vi "KE622x -- Get Buf Size.vi"(0 "Resource In":refnum<visa-resource-name>, 1 "Check For SCPI Errors? (T)":bool=TRUE, 11 "error in (no error)":errorcluster) -> (4 "Resource Out (dupl)":refnum<visa-resource-name>, 8 "Buffer Size (Num Readings)":T1 min=1 max=65536 step=1, 15 "error out":errorcluster)   [LabVIEW 2019, in "Keithley 622x.lvlib"]
uses:
  Keithley 622x.lvlib
  Typedefs/KE622x -- Trace Buf Size.ctl
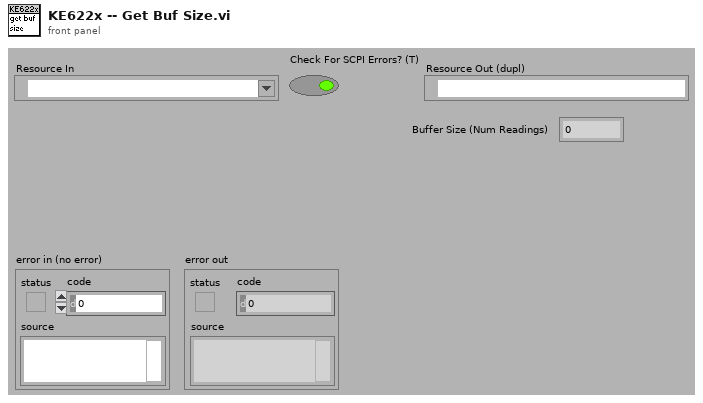
[diagram p1: front panel]
types:
  T1 = typedef "Keithley 622x.lvlib/KE622x -- Trace Buf Size.ctl" = u32
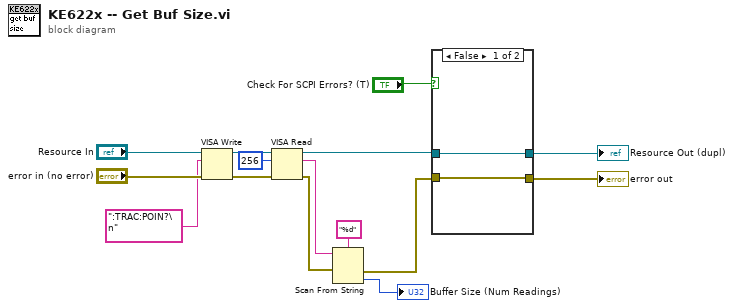
[diagram p0: block diagram]
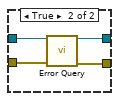
[diagram p2: hidden frame]
diagram:
  n1 = VISA Write(VISA resource name="Resource In", write buffer=":TRAC:POIN?\n" ("format string"), error in (no error)="error in (no error)") -> (VISA resource name out=w15:refnum<visa-resource-name>, error out=w14:errorcluster)  [unwired: 1 out]
  n2 = VISA Read(VISA resource name=w15, byte count=u32 256, error in (no error)=w14) -> (VISA resource name out=w5:refnum<visa-resource-name>, read buffer=w9:string, error out=w7:errorcluster)  [unwired: 1 out]
  n3 = Scan From String(format string="%d", input string=w9, error in=w7) -> (error out=w6:errorcluster, output 1=→"Buffer Size (Num Readings)":T1)  [unwired: 2 in, 2 out]
  n4 = case shown="False" "Check For SCPI Errors? (T)" {
    tunnel: w5 -> [w17 w21]
    tunnel: w6 -> [w16 w20]
    tunnel: [w16 w19] -> w1
    tunnel: [w17 w18] -> w2
    frame False {
    }
    frame True {
      n5 = call "Error Query.vi"("VISA Resource In"=w21, "error in (no error)"=w20) -> ("VISA Resource Out (dupl)"=w18:refnum<visa-resource-name>, "error out"=w19:errorcluster)  [unwired: 10 in, 2 out]
    }
  }
  "Resource Out (dupl)" <- w2
  "error out" <- w1
